vi "Rotate_2D_Peregrine.vi"(8 "Angle(rad)":dbl, 10 "Y axis coordinate in":dbl, 11 "X axis coordinate in":dbl) -> (2 "Y axis coordinate out":dbl, 3 "X axis coordinate out":dbl)   [LabVIEW 2019]
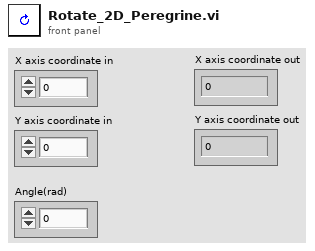
[diagram p1: front panel]
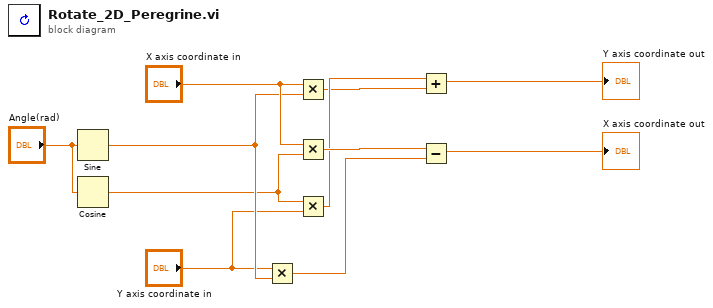
[diagram p0: block diagram]
diagram:
  n1 = Sine(x="Angle(rad)") -> (sin(x)=w7:dbl)
  n2 = Cosine(x="Angle(rad)") -> (cos(x)=w5:dbl)
  n3 = Multiply(x="Y axis coordinate in", y=w7) -> (x*y=w10:dbl)
  n4 = Multiply(x="X axis coordinate in", y=w7) -> (x*y=w3:dbl)
  n5 = Multiply(x="X axis coordinate in", y=w5) -> (x*y=w11:dbl)
  n6 = Multiply(x=w5, y="Y axis coordinate in") -> (x*y=w4:dbl)
  n7 = Add(x=w4, y=w3) -> (x+y=→"Y axis coordinate out":dbl)
  n8 = Subtract(x=w11, y=w10) -> (x-y=→"X axis coordinate out":dbl)
